vi "ep_Torque Check Error (1 Chan).vi"(0 "signal":waveform(dbl), 2 "reset? (F)":bool, 5 "speed [RPM]":dbl, 7 "nominal frequency":enum16{"50 Hz", "60 Hz"}(ring), 9 "motor information":T3, 11 "error in (no error)":errorcluster, 12 "initial conditions":T1, 13 "stator resistance [ohms]":dbl) -> (8 "information":T2, 14 "final conditions":T1, 15 "error out":errorcluster)   [LabVIEW 2014, in "NI_EP_Motor Monitoring.lvlib"]
uses:
  <vilib>/addons/Electrical Power/Motor Monitoring/NI_EP_Motor Monitoring.lvlib
  <vilib>/addons/Electrical Power/Motor Monitoring/subVIs/ep_Initial Conditions for Air Gap.ctl
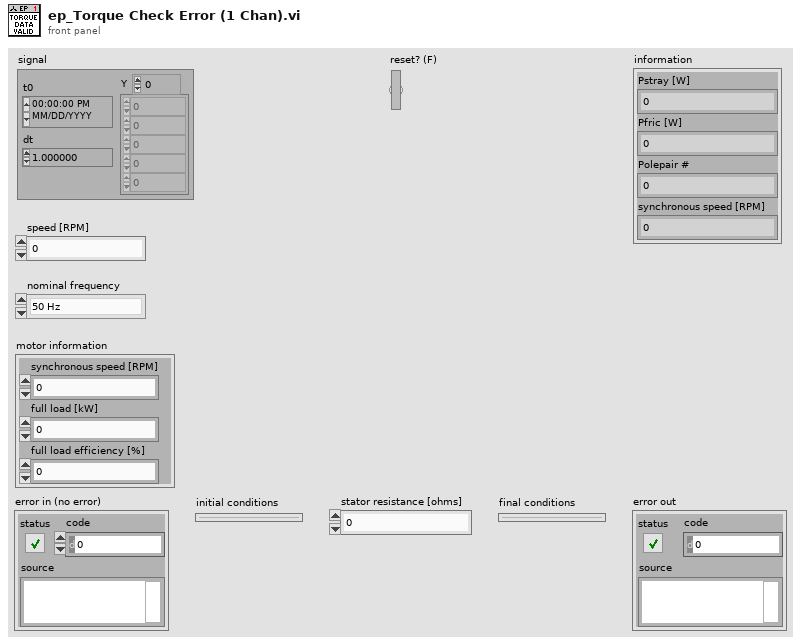
[diagram p1: front panel]
types:
  T1 = typedef "NI_EP_Motor Monitoring.lvlib/ep_Initial Conditions for Air Gap.ctl" = cluster{"integration state in A":cluster{"initial value":dbl, "initial integration":dbl}, "integration state in B":cluster{"initial value":dbl, "initial integration":dbl}, "integrated state A":dbl[], "integrated state B":dbl[], "previous length":i32, "loss and polepair":cluster{"Pstray [W]":dbl, "Pfric [W]":dbl, "Polepair #":i32, "synchronous speed [RPM]":dbl}, "expected timestamp":timestamp}
  T2 = cluster{"Pstray [W]":dbl, "Pfric [W]":dbl, "Polepair #":i32, "synchronous speed [RPM]":dbl}
  T3 = cluster{"synchronous speed [RPM]":dbl, "full load [kW]":dbl, "full load efficiency [%]":dbl}
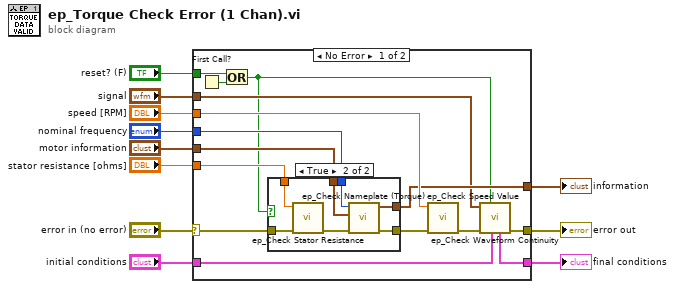
[diagram p0: block diagram]
diagram:
  n1 = case shown="No Error" "error in (no error)" {
    selector: "error in (no error)" -> [w21 w35]
    tunnel: [w17 w35] -> w10
    tunnel: "speed [RPM]" -> [w20 _]
    tunnel: "motor information" -> [w26 _]
    tunnel: "nominal frequency" -> [w25 _]
    tunnel: "stator resistance [ohms]" -> [w24 _]
    tunnel: "reset? (F)" -> [w22 _]
    tunnel: [w19 _] -> w5
    tunnel: "initial conditions" -> [w16 _]
    tunnel: [w15 _] -> w2
    tunnel: "signal" -> [w14 _]
    frame No Error {
      n2 = First Call?() -> (First Call?: T/F=w23:bool)
      n3 = Or(x=w22, y=w23) -> (x .or. y?=w13:bool)
      n4 = case shown="True" w13 {
        tunnel: w26 -> [_ w34]
        tunnel: w25 -> [_ w33]
        tunnel: w24 -> [_ w32]
        tunnel: [w27 w29] -> w12
        tunnel: w21 -> [w27 w31]
        tunnel: [_ w28] -> w19
        frame False {
        }
        frame True {
          n5 = call <vilib>:"ep_Check Stator Resistance.vi"("error in (no error)"=w31, "stator resistance  [ohms]"=w32) -> ("error out"=w30:errorcluster)  [unwired: 9 in]
          n6 = call <vilib>:"ep_Check Nameplate (Torque).vi"("error in (no error)"=w30, "motor information"=w34, "nominal frequency"=w33) -> ("error out"=w29:errorcluster, "information"=w28:T2)  [unwired: 7 in]
        }
      }
      n7 = call <vilib>:"ep_Check Speed Value.vi"("error in (no error)"=w12, "speed [RPM]"=w20) -> ("error out"=w18:errorcluster)  [unwired: 9 in]
      n8 = call <vilib>:"ep_Check Waveform Continuity.vi"("initial conditions"=w16, "reset? (F)"=w13, "error in (no error)"=w18, "signal"=w14) -> ("error out"=w17:errorcluster, "final conditions"=w15:T1)  [unwired: 6 in]
    }
    frame Error {
    }
  }
  "error out" <- w10
  "information" <- w5
  "final conditions" <- w2
